vi "Enter Calibration Code.vi"(4 "Calibration Code":T2(ring), 7 "output cluster":T3, 11 "CalStatus":T1(ring)) -> (3 "NewCalStatus":T1(ring))   [LabVIEW 2015]
uses:
  Controls/Cal Refs.ctl
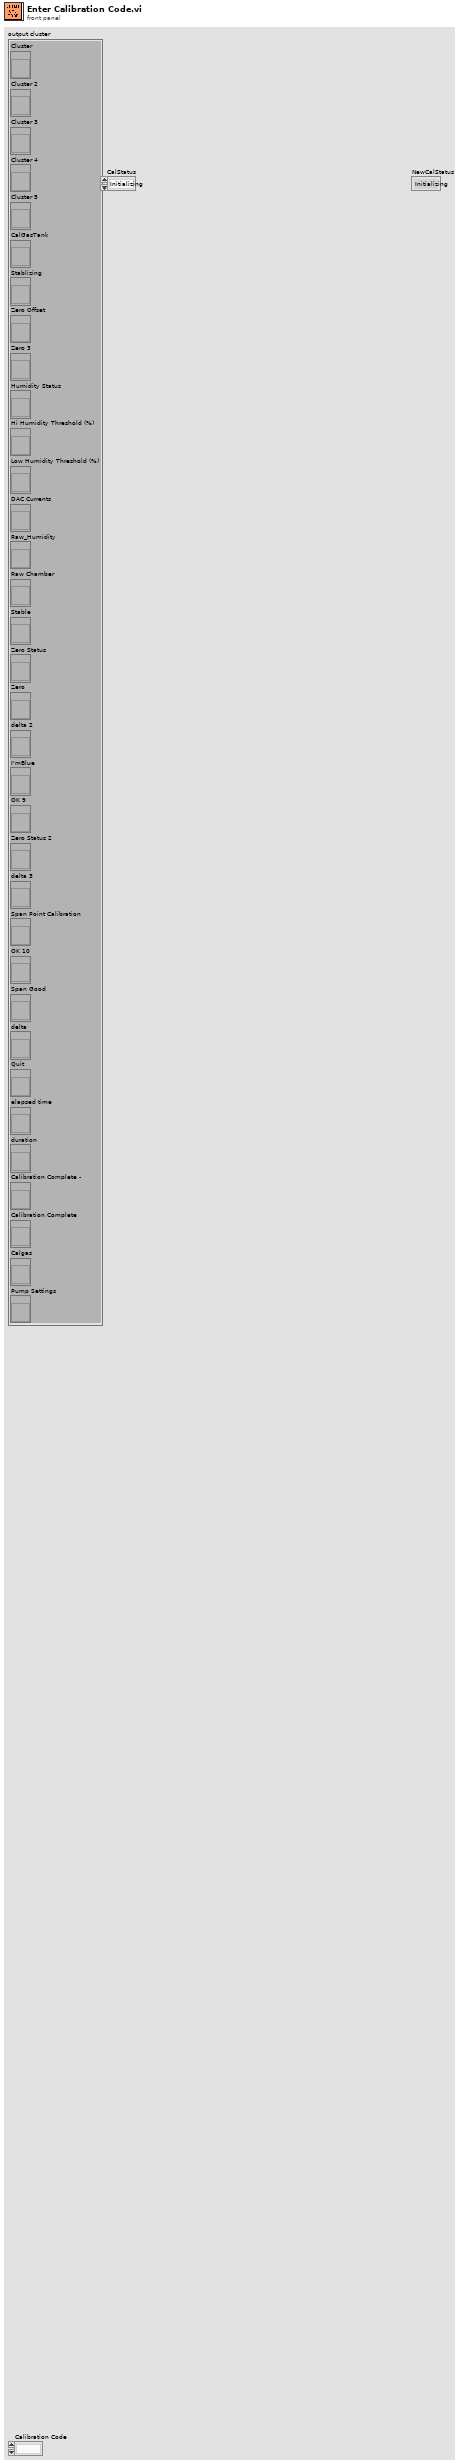
[diagram p1: front panel]
types:
  T1 = enum32{"Initializing", "Enter CO2 Value", "Enter Calibration Code", "Reading Calibration Data", "Stablizing", "Calculating Target Voltages", "Setting Zero Point", "Setting High Point", "Setting Span Point", "Calculating Gain & Offset", "Storing Calibration Coefficients", "Calibration Complete"}
  T2 = enum8{"", "<User Defined>", "11111 - default", "22222 - MM_1_NS", "33333 - MM_2_S"}
  T3 = typedef "Cal Refs.ctl" = cluster{"Cluster":refnum<vi>, "Cluster 2":refnum<vi>, "Cluster 3":refnum<vi>, "Cluster 4":refnum<vi>, "Cluster 5":refnum<vi>, "CalGasTank":refnum<vi>, "Stablizing":refnum<vi>, "Zero Offset":refnum<vi>, "Zero 3":refnum<vi>, "Humidity Status":refnum<vi>, "Hi Humidity Threshold (%)":refnum<vi>, "Low Humidity Threshold (%)":refnum<vi>, "DAC Currents":refnum<vi>, "Raw_Humidity":refnum<vi>, "Raw Chamber":refnum<vi>, "Stable":refnum<vi>, "Zero Status":refnum<vi>, "Zero":refnum<vi>, "delta 2":refnum<vi>, "I'mBlue":refnum<vi>, "OK 9":refnum<vi>, "Zero Status 2":refnum<vi>, "delta 3":refnum<vi>, "Span Point Calibration":refnum<vi>, "OK 10":refnum<vi>, "Span Good":refnum<vi>, "delta":refnum<vi>, "Quit":refnum<vi>, "elapsed time":refnum<vi>, "duration":refnum<vi>, "Calibration Complete -":refnum<vi>, "Calibration Complete":refnum<vi>, "Calgas":refnum<vi>, "Pump Settings":refnum<vi>}
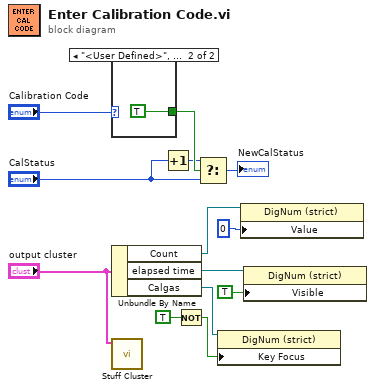
[diagram p0: block diagram]
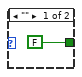
[diagram p2: hidden frame]
diagram:
  n1 = case shown="\"<User Defined>\", Default" "Calibration Code" {
    tunnel: [FALSE TRUE] -> w4
    frame "" {
    }
    frame "<User Defined>", Default {
    }
  }
  n2 = Unbundle By Name("output cluster") -> ("Count"=w9:refnum<vi>, "elapsed time"=w12:refnum<vi>, "Calgas"=w13:refnum<vi>)
  n3 = call "Stuff Cluster.vi"("output cluster"="output cluster") -> ()  [unwired: 10 in, 1 out]
  n4 = Increment(x="CalStatus") -> (x+1=w3:T1)
  n5 = Not(x=TRUE ("Key Focus")) -> (.not. x?=w7:bool)
  n6 = Select(t=w3, s=w4, f="CalStatus") -> (s? t:f=→"NewCalStatus":T1)
  n7 = property on="Property Node" class="DigNum (strict)"(reference=w13, "Key Focus"=w7) -> ()  [unwired: 1 in, 2 out]
  n8 = property class="DigNum (strict)"(reference=w9, "Value"=u8 0) -> ()  [unwired: 1 in, 2 out]
  n9 = property on="Property Node" class="DigNum (strict)"(reference=w12, "Visible"=TRUE) -> ()  [unwired: 1 in, 2 out]
